vi "Set Initialization Data - Worker A.vi"(8 "error in":errorcluster, 11 "Head Worker in":refnum<class "Head Worker.lvclass">) -> (0 "error out":errorcluster, 3 "Head Worker out":refnum<class "Head Worker.lvclass">)   [LabVIEW 2017, in "Head Worker.lvclass"]
doc: "In this VI you can set the initialization data of a statically-linked subWorker."
uses:
  Head Worker.lvclass
  Worker A/Initialization Data.ctl
  Worker A/Response Cases.ctl
  Head Worker.lvclass/Head Worker.ctl
  Worker A/Worker A.lvclass
  C:/Program Files (x86)/National Instruments/LabVIEW 2017/vi.lib/addons/_Workers/Library/Classes/Worker/Worker.lvclass
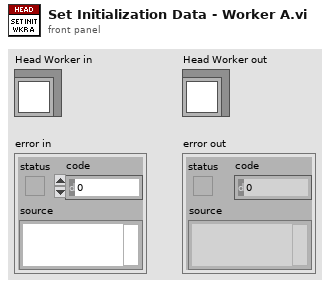
[diagram p1: front panel]
types:
  T1 = typedef "Worker A.lvclass/Initialization Data.ctl" = cluster{"Response Cases":T2}
  T2 = typedef "Worker A.lvclass/Response Cases.ctl" = cluster{"Placeholder - Can be deleted":string}
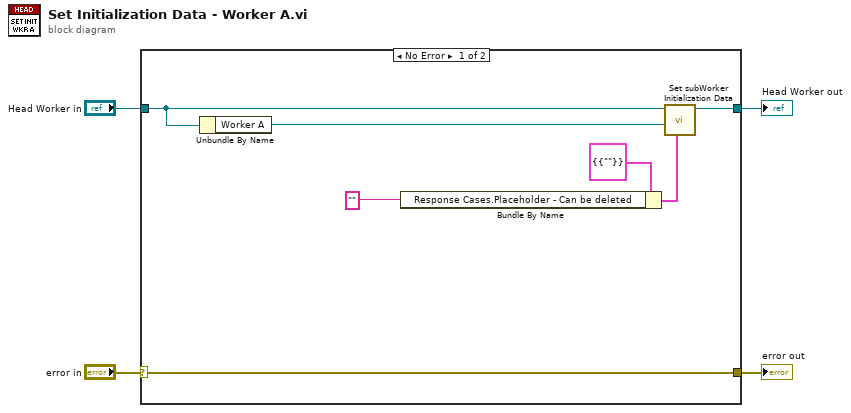
[diagram p0: block diagram]
diagram:
  n1 = case shown="No Error" "error in" {
    selector: "error in" -> [w11 w13]
    tunnel: [w11 w13] -> w3
    tunnel: [w9 w12] -> w2
    tunnel: "Head Worker in" -> [w8 w12]
    frame No Error {
      n2 = Unbundle By Name(w8) -> ("Worker A"=w10:refnum<class "Worker A.lvclass">)
      n3 = Bundle By Name(cluster=T1 {"Response Cases"={"Placeholder - Can be deleted"=""}} ("Initialization Data"), "Response Cases.Placeholder - Can be deleted"="") -> (w6:T1)
      n4 = call-dynamic "Set subWorker Initialization Data.vi"("Initialization Data"=w6, "subWorker"=w10, "Worker"=w8) -> ("Worker out"=w9:refnum<class "Head Worker.lvclass">)  [unwired: 8 in]
    }
    frame Error {
    }
  }
  "error out" <- w3
  "Head Worker out" <- w2
